vi "IsHotGoalDB.vi"(8 "error in":errorcluster, 9 "DBHot?":string="Boolean", 10 "DBFinished?":string="Boolean", 11 "DBStart":string="Boolean") -> (0 "error out":errorcluster, 2 "Hot?":bool)   [LabVIEW 2013]
doc: "IsHotGoalDB determines whether or not the goal is hot. Image processing is done on the laptop (through the DB).\n-DBStart: the name of the DB boolean control that starts image processing. IsHotGoalDB writes to this to signal the DB to start.\n-DBFinished?: the name of the DB boolean indicator that indicates when the DB is done processing.\n-DBHot?: the name of the DB boolean indicator that indicates whether the goal is hot."
panel:
  in  "milliseconds to wait":u32=20
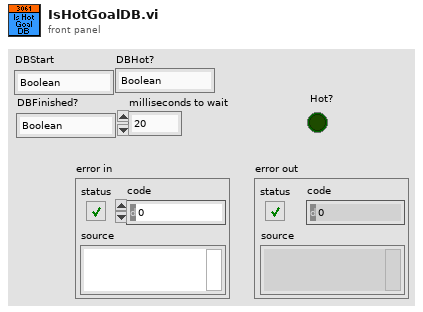
[diagram p1: front panel]
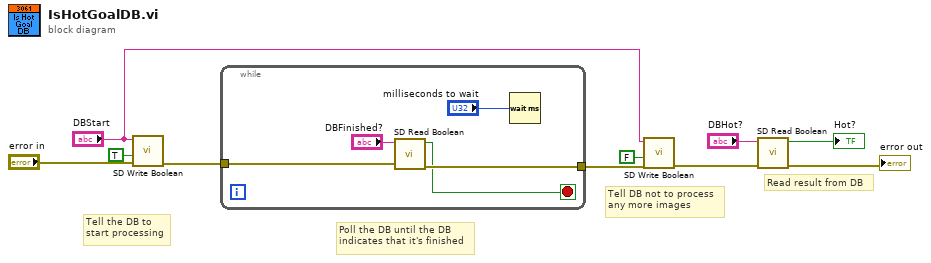
[diagram p0: block diagram]
diagram:
  # "Tell DB not to process\nany more images"
  # "Read result from DB"
  # "Poll the DB until the DB\nindicates that it's finished"
  # "Tell the DB to\nstart processing"
  n1 = call <vilib>:"SD Write Boolean.vi"("error in"="error in", "Boolean"=TRUE, "Name"="DBStart") -> ("error out"=w9:errorcluster)  [unwired: 7 in, 1 out]
  n2 = while {
    tunnel: w9 -> [w14]
    tunnel: [w13] -> w3
    stop <- w12 stop-if-true
    n3 = call <vilib>:"SD Read Boolean.vi"("error in"=w14, "Name"="DBFinished?") -> ("error out"=w13:errorcluster, "Boolean"=w12:bool)  [unwired: 7 in, 1 out]
    n4 = Wait (ms)(milliseconds to wait="milliseconds to wait") -> ()  [unwired: 1 out]
  }
  n5 = call <vilib>:"SD Write Boolean.vi"("error in"=w3, "Boolean"=FALSE, "Name"="DBStart") -> ("error out"=w2:errorcluster)  [unwired: 7 in, 1 out]
  n6 = call <vilib>:"SD Read Boolean.vi"("error in"=w2, "Name"="DBHot?") -> ("error out"=→"error out":errorcluster, "Boolean"=→"Hot?":bool)  [unwired: 7 in, 1 out]
